vi "Export FIR Coefficients to Xilinx COE File.vi"() -> ()   [LabVIEW 2023]
doc: "Demonstrates how to export integer finite impulse response (FIR) coefficients of a filter from a text file that you generated using the DFD Save to Text File VI. This example also demonstrates how to use the exported coefficients to build a .coe file. To create the .coe file, specify a valid path to the .coe file in the <B>COE File Path</B> input. You can load the .coe file using the the Xilinx CORE Generator (TM).\n\nXilinx (R) is the registered trademark of Xilinx, Inc."
uses:
  <vilib>/addons/Digital Filter Design/FXPModel.llb/DFD FXP Quantize Coef (Easy).vi
  <vilib>/addons/Digital Filter Design/FilterLib.llb/DFD Save Filter to Text File.vi
  <vilib>/addons/Digital Filter Design/NI_DigFilterLicensed.lvlib
panel:
  in  "Coefficient Type":T1(ring)
  out "Error Message":string
  in  "COE File Path":path
  out "COE Text":string
  in  "Text Filter File Path":path
  in  "Coefficients b/v Word Length":i16=16
  # "Select Help>>Show Context Help and move the cursor over the VI icon for more information."
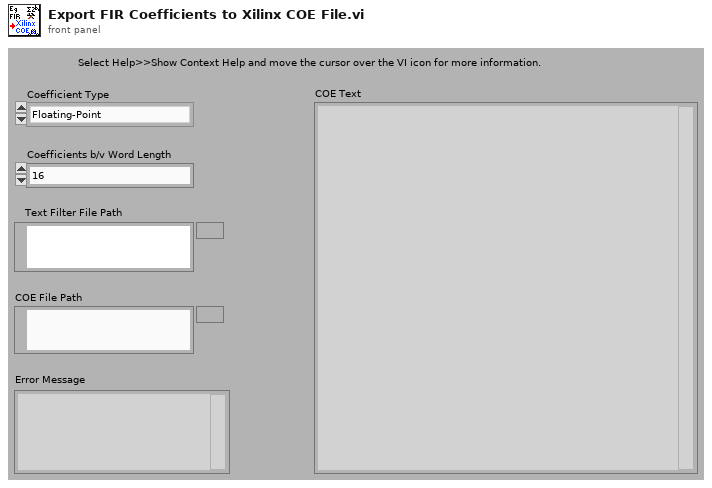
[diagram p1: front panel]
types:
  T1 = enum16{"Floating-Point", "Fixed-Point", "Integer"}
  T2 = typedef "NI_DigFilterLicensed.lvlib/DFD Filter Obj.ctl" = cluster{"mSRate_Fs":dbl, "mSRate_Version":string, "mSRate_Comments":string, "mSRate_OrgCoef":T3, "mSRate_CurCoef":T3, "mSRate_Quantized?":bool, "mSRate_QCoef":T3, "mSRate_QSettings":T5[], "mSRate_Order":i32, "mSRate_Scaling":cluster{"mSRate_ScaleByPowerOf2?":bool, "mSRate_ScaleType":T7}}
  T3 = typedef "NI_DigFilterLicensed.lvlib/DFD Filter Coef.ctl" = cluster{"type":T4, "gain":dbl, "coef a (k)":dbl[], "coef b (v)":dbl[]}
  T4 = typedef "NI_DigFilterLicensed.lvlib/DFD Filter Structure Type Selector.ctl" = enum16{"Undefined", "FIR Direct Form", "FIR Direct Form Transposed", "FIR Symmetric", "FIR Antisymmetric", "IIR Direct Form I", "IIR Direct Form I Transposed", "IIR Direct Form II", "IIR Direct Form II Transposed", "IIR Cascaded Second Order Sections Form I", "IIR Cascaded Second Order Sections Form I Transposed", "IIR Cascaded Second Order Sections Form II", "IIR Cascaded Second Order Sections Form II Transposed", "Lattice Allpass (basic sections)", "Lattice Allpass (one multiplier sections)", "Lattice Allpass (normalized sections)", "Lattice AR (basic sections)", "Lattice AR (one multiplier sections)", "Lattice AR (normalized sections)", "Lattice MA (minimum phase)", "Lattice MA (maximum phase)", "Lattice ARMA (basic sections)", "Lattice ARMA (one multiplier sections)", "Lattice ARMA (normalized sections)"}
  T5 = typedef "NI_DigFilterLicensed.lvlib/dfd_Internal Quantization Settings.ctl" = cluster{"source":T6, "wl":i16, "iwl":i16, "overflow mode":enum16{"Saturation", "Wrap"}, "rounding mode":enum16{"Nearest", "Truncation"}, "signed?":bool}
  T6 = typedef "NI_DigFilterLicensed.lvlib/dfd_Internal Quantization Srcs.ctl" = u16
  T7 = typedef "NI_DigFilterLicensed.lvlib/DFD Coef Norm Type.ctl" = enum16{"No Norm", "Time Domain 1-Norm", "Time Domain 2-Norm", "Time Domain Inf-Norm"}
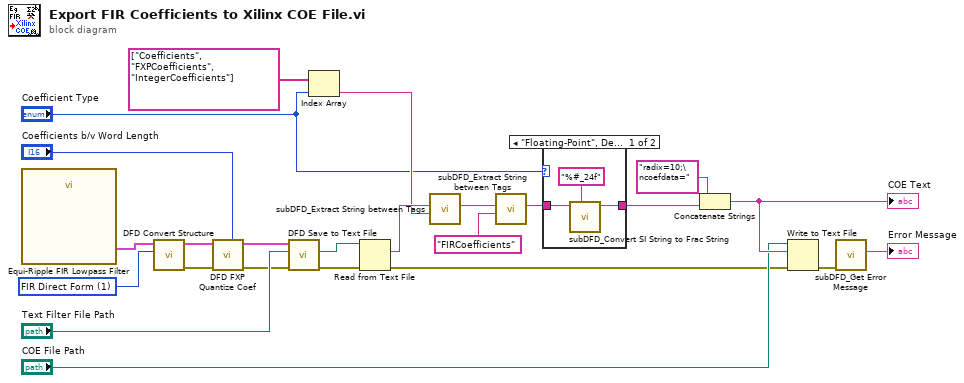
[diagram p0: block diagram]
diagram:
  w8 = u16 1 items=["FIR Direct Form"=1, "FIR Direct Form Transposed"=2, "FIR Symmetric"=3, "FIR Antisymmetric"=4, "IIR Direct Form I"=5, "IIR Direct Form I Transposed"=6, "IIR Direct Form II"=7, "IIR Direct Form II Transposed"=8, "IIR Cascaded Second-Order Sections Form I"=9, "IIR Cascaded Second-Order Sections Form I Transposed"=10, "IIR Cascaded Second-Order Sections Form II"=11, "IIR Cascaded Second-Order Sections Form II Transposed"=12, "Lattice Allpass (basic sections)"=13, "Lattice Allpass (one multiplier sections)"=14, "Lattice Allpass (normalized sections)"=15, "Lattice AR (basic sections)"=16, "Lattice AR (one multiplier sections)"=17, "Lattice AR (normalized sections)"=18, "Lattice MA (minimum phase)"=19, "Lattice MA (maximum phase)"=20, "Lattice ARMA (basic sections)"=21, "Lattice ARMA (one multiplier sections)"=22, "Lattice ARMA (normalized sections)"=23] ("target structure")
  n1 = call "Equi-Ripple FIR Lowpass Filter"() -> ("filter out"=w1:T2)  [unwired: 1 in, 10 out]
  n2 = call <vilib>:"DFD Convert Structure.vi"("target structure"=w8, "filter in"=w1) -> ("error out"=w11:errorcluster, "filter out"=w12:T2)  [unwired: 1 in, 7 out]
  n3 = call-poly <vilib>:"DFD FXP Quantize Coef.vi"("coefficients b/v word length"="Coefficients b/v Word Length", "error in (no error)"=w11, "filter in"=w12) -> ("error out"=w22:errorcluster, "filter out"=w24:T2)  [unwired: 2 in, 5 out]
  n4 = call-poly <vilib>:"DFD Save to Text File.vi"("error in (no error)"=w22, "file path in"="Text Filter File Path", "filter in"=w24) -> ("error out"=w20:errorcluster, "file path out"=w21:path)  [unwired: 1 in, 6 out]
  n5 = Index Array(array=string[] ["Coefficients", "FXPCoefficients", "IntegerCoefficients"], index="Coefficient Type") -> (element=w6:string)
  n6 = Read from Text File(file (use dialog)=w21, error in=w20) -> (text=w19:string, error out=w4:errorcluster)  [unwired: 4 out]
  n7 = call "subDFD_Extract String between Tags.vi"("tag"=w6, "original string"=w19) -> ("extracted string"=w10:string)  [unwired: 1 in, 8 out]
  n8 = call "subDFD_Extract String between Tags.vi"("tag"="FIRCoefficients", "original string"=w10) -> ("extracted string"=w3:string)  [unwired: 1 in, 8 out]
  n9 = case shown="\"Floating-Point\", Default" "Coefficient Type" {
    tunnel: w3 -> [w27 w28]
    tunnel: [w26 w28] -> w2
    frame "Floating-Point", Default {
      n10 = call "subDFD_Convert SI String to Frac String.vi"("format string"="%#_24f", "SI string in"=w27) -> ("Fractional string out"=w26:string)  [unwired: 9 out]
    }
    frame "Integer" {
    }
  }
  n11 = Concatenate Strings("radix=10;\ncoefdata=", w2) -> (w17:string)
  "COE Text" <- w17
  n12 = Write to Text File(file (use dialog)="COE File Path", text=w17, error in=w4) -> (error out=w15:errorcluster)  [unwired: 3 out]
  n13 = call <vilib>:"subDFD_Get Error Message.vi"("error in (no error)"=w15) -> ("Error Message"=→"Error Message":string)  [unwired: 10 out]
